vi "Copy Blob.vi"(5 "Destination Blob":string, 7 "Destination Container":string, 8 "error in (no error)":errorcluster, 9 "Source Blob":string, 10 "Source Container":string, 11 "Azure Session in":refnum<class "Session.lvclass">) -> (0 "error out":errorcluster, 2 "Copy ID":string, 3 "Azure Session out":refnum<class "Session.lvclass">)   [LabVIEW 2015, in "NI_Azure_Blob.lvlib"]
doc: "Copies a source blob to a destination blob in the current storage account."
uses:
  NI_Azure_Blob.lvlib
  Core/Session/Session.lvclass
  Core/Name Value Pair.ctl
  Core/Session/Session.lvclass/Session.ctl
  Core/Session/Read Credentials.vi
  Core/Session/Write Request Headers.vi
  Core/Session/Write URL Suffix.vi
  Core/Session/Write HTTP Verb.vi
  Core/NI_Azure_Core.lvlib
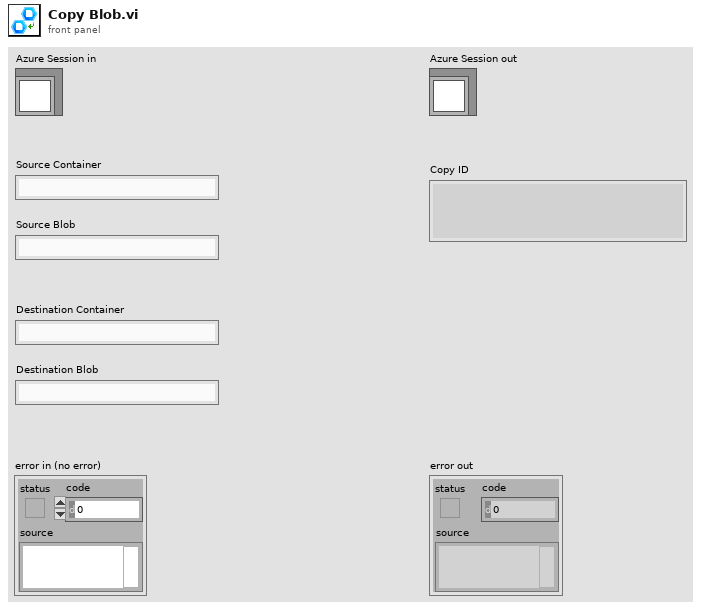
[diagram p1: front panel]
types:
  T1 = typedef "NI_Azure_Core.lvlib/Name Value Pair.ctl" = cluster{"name":string, "value":string}
  T2 = typedef "NI_Azure_Core.lvlib/Session.lvclass/Azure Credentials.ctl" = cluster{"Storage Account Name":string, "Access Key":string}
  T3 = typedef "NI_Azure_Core.lvlib/Response.ctl" = cluster{"Headers":string, "Body":string}
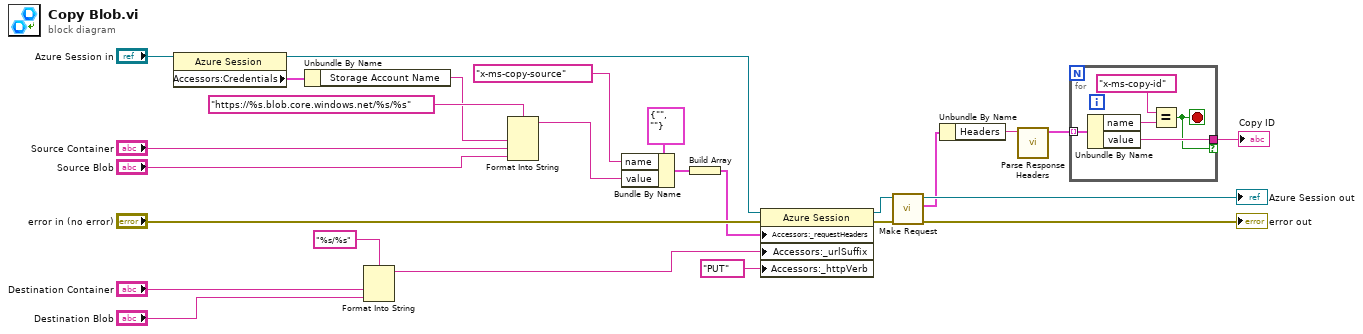
[diagram p0: block diagram]
diagram:
  n1 = property class="Azure Session"(reference="Azure Session in") -> (reference out=w7:refnum<class "Session.lvclass">, "Accessors:Credentials"=w19:T2)  [unwired: 1 in, 1 out]
  n2 = Unbundle By Name(w19) -> ("Storage Account Name"=w12:string)
  n3 = Format Into String(format string="%s/%s", "Destination Container", "Destination Blob") -> (resulting string=w6:string)  [unwired: 2 in, 1 out]
  n4 = Format Into String(format string="https://%s.blob.core.windows.net/%s/%s" ("url"), w12, "Source Container", "Source Blob") -> (resulting string=w13:string)  [unwired: 2 in, 1 out]
  n5 = Bundle By Name(cluster=T1 {"name"="", "value"=""} ("Name Value Pair"), "name"="x-ms-copy-source" ("header"), "value"=w13) -> (w15:T1)
  n6 = Build Array(w15) -> (w8:T1[])
  n7 = property class="Azure Session"(reference=w7, error in="error in (no error)", "Accessors:_requestHeaders"=w8, "Accessors:_urlSuffix"=w6, "Accessors:_httpVerb"="PUT" ("HTTP-Verb")) -> (reference out=w9:refnum<class "Session.lvclass">, error out=w10:errorcluster)
  n8 = call "Make Request.vi"("error in (no error)"=w10, "Session in"=w9) -> ("error out"=→"error out":errorcluster, "Response"=w4:T3, "Session out"=→"Azure Session out":refnum<class "Session.lvclass">)  [unwired: 7 in]
  n9 = Unbundle By Name(w4) -> ("Headers"=w3:string)
  n10 = call "Parse Response Headers.vi"("String"=w3) -> ("Response Headers"=w2:T1[])  [unwired: 10 in]
  n11 = for {
    tunnel: w2 -> [w31] mode=indexing
    tunnel: [w28] -> w1 if=w27
    stop <- w27 stop-if-true
    n12 = Unbundle By Name(w31) -> ("name"=w30:string, "value"=w28:string)
    n13 = Equal?(x="x-ms-copy-id", y=w30) -> (x = y?=w27:bool)
  }
  "Copy ID" <- w1
